vi "UHR-Fleezers Control (host) - Lorentz v3.vi"() -> ()   [LabVIEW 2014] (continued)
            n1301 = Unbundle By Name(w2020) -> ("Set 1"=w2019:dbl, "Set 2"=w2018:dbl)
            n1302 = Unbundle By Name(w2017) -> ("Set 1"=w2016:bool, "Set 2"=w2015:bool)
            n1303 = Select(t=w2013, s=w2016, f=w2019) -> (s? t:f=w2011:dbl)
            n1304 = Select(t=w2012, s=w2015, f=w2018) -> (s? t:f=w2010:dbl)
            n1305 = Bundle By Name(cluster=w2020, "Set 1"=w2011, "Set 2"=w2010) -> (w2008:cluster{"Set 1":dbl, "Set 2":dbl})
            n1306 = local write "Setpoints (V)"(w2008) -> ()
            n1307 = Multiply(x=3276.7, y=w2008) -> (x*y=w2009:cluster{"Set 1":dbl, "Set 2":dbl})
            n1308 = To Word Integer(number=w2009) -> (16bit integer=w2021:cluster{"Set 1":i16, "Set 2":i16})
          }
        }
        n1309 = Unbundle By Name(w1993) -> ("Set 1"=w1992:i16, "Set 2"=w1991:i16)
        n1310 = xnode "Read/Write Control"("FPGA VI Reference In"=w1990, "error in"=w1989, "FB Setpoint Set 1"=w1992, "FB Setpoint Set 2"=w1991) -> ("error out"=w1988:errorcluster)  [unwired: 1 out]
      }
      event "+ phase (GI)", "- phase (GI)", "+ phase (GI) 2", "- phase (GI) 2", "+ phase (RI)", "- phase (RI)", "+ phase (Green FB)", "- phase (Green FB)", "- phase (BI AO)", "+ phase (BI AO)", "- phase (BI DO)", "+ phase (BI DO)": Value Change {
        n1311 = event-data() -> ()  [unwired: 7 out]
        n1312 = Or(x="+ phase (GI)", y="- phase (GI)") -> (x .or. y?=w2057:bool)
        n1313 = Negate(x="Phase adj. (GI)") -> (-x=w2062:i16)
        n1314 = Select(t=w2062, s="+ phase (GI)", f="Phase adj. (GI)") -> (s? t:f=w2061:i16)
        n1315 = Or(x="+ phase (GI) 2", y="- phase (GI) 2") -> (x .or. y?=w2048:bool)
        n1316 = Negate(x="Phase adj. (GI) 2") -> (-x=w2053:i16)
        n1317 = Select(t=w2053, s="+ phase (GI) 2", f="Phase adj. (GI) 2") -> (s? t:f=w2049:i16)
        n1318 = Negate(x="Phase adj. (RI)") -> (-x=w2047:i16)
        n1319 = Or(x="+ phase (RI)", y="- phase (RI)") -> (x .or. y?=w2043:bool)
        n1320 = Select(t=w2047, s="+ phase (RI)", f="Phase adj. (RI)") -> (s? t:f=w2042:i16)
        n1321 = Or(x="+ phase (Green FB)", y="- phase (Green FB)") -> (x .or. y?=w2036:bool)
        n1322 = Negate(x="Phase adj. (Green FB)") -> (-x=w2041:i16)
        n1323 = Select(t=w2041, s="+ phase (Green FB)", f="Phase adj. (Green FB)") -> (s? t:f=w2037:i16)
        n1324 = Negate(x="Phase adj. (BI AO)") -> (-x=w2035:i16)
        n1325 = Or(x="+ phase (BI AO)", y="- phase (BI AO)") -> (x .or. y?=w2025:bool)
        n1326 = Select(t=w2035, s="+ phase (BI AO)", f="Phase adj. (BI AO)") -> (s? t:f=w2027:i16)
        n1327 = Negate(x="Phase adj. (BI DO)") -> (-x=w2031:i16)
        n1328 = Or(x="+ phase (BI DO)", y="- phase (BI DO)") -> (x .or. y?=w2024:bool)
        n1329 = Select(t=w2031, s="+ phase (BI DO)", f="Phase adj. (BI DO)") -> (s? t:f=w2026:i16)
        n1330 = xnode "Read/Write Control"("FPGA VI Reference In"=w2023, "Phase count adjustment (GI)"=w2061, "Phase count adjustment (GI) 2"=w2049, "Phase count adjustment (RI)"=w2042, "Phase count adjustment (Green FB)"=w2037, "Phase count adjustment (BI AO)"=w2027, "Phase count adjustment (BI D)"=w2026) -> ("FPGA VI Reference Out"=w2059:T36, "error out"=w2060:errorcluster)  [unwired: 1 in]
        n1331 = xnode "Read/Write Control"("FPGA VI Reference In"=w2059, "error in"=w2060, "+ phase (GI)"=w2057, "+ phase (GI) 2"=w2048, "+ phase (RI)"=w2043, "+ phase (Green FB)"=w2036, "+ phase (BI AO)"=w2025, "+ phase (BI D)"=w2024) -> ("error out"=w2058:errorcluster)  [unwired: 1 out]
      }
      event "Green Laser ON/OFF", "Red Laser ON/OFF", "Blue Laser ON/OFF": Value Change {
        # "This loop shouldn't be initialized.  The main 'laser ON' settings should dominate and set the others."
        n1332 = event-data() -> ()  [unwired: 7 out]
        n1333 = property on="Red Laser ON" class="Bool (strict)"("Val(Sgnl)"="Red Laser ON/OFF") -> ()  [unwired: 2 in, 2 out]
        n1334 = property on="Blue Laser ON" class="Bool (strict)"("Val(Sgnl)"="Blue Laser ON/OFF") -> ()  [unwired: 2 in, 2 out]
        n1335 = property on="Green Laser ON" class="Bool (strict)"("Val(Sgnl)"="Green Laser ON/OFF") -> ()  [unwired: 2 in, 2 out]
      }
      event "Laser interlacing mode", "Green Laser ON", "Red Laser ON", "Blue Laser ON": Value Change {
        n1336 = event-data() -> ()  [unwired: 7 out]
        n1337 = local write "Green Laser ON/OFF"("Green Laser ON") -> ()
        n1338 = local write "Blue Laser ON/OFF"("Blue Laser ON") -> ()
        n1339 = local write "Red Laser ON/OFF"("Red Laser ON") -> ()
        n1340 = case shown="False" "Green Laser ON" {
          tunnel: "Laser interlacing mode" -> [_ w2123]
          tunnel: [enum32{"Laser ON", "Laser OFF", "Interlace"}."Laser OFF" ("Green laser mode") w2123] -> w2099
          tunnel: [FALSE w2119] -> w2098
          frame False {
          }
          frame True {
            n1341 = local read "Green FB On/Off"() -> (w2120:bool)
            n1342 = Equal?(x=w2123, y=enum32{"Laser ON", "Laser OFF", "Interlace"}."Interlace") -> (x = y?=w2121:bool)
            n1343 = And(x=w2121, y=w2120) -> (x .and. y?=w2119:bool)
          }
        }
        n1344 = case shown="True" "Red Laser ON" {
          tunnel: "Laser interlacing mode" -> [_ w2116]
          tunnel: [enum32{"Laser ON", "Laser OFF", "Interlace"}."Laser OFF" ("Green laser mode") w2116] -> w2095
          tunnel: [FALSE w2112] -> w2094
          frame False {
          }
          frame True {
            n1345 = local read "Red FB On/Off"() -> (w2113:bool)
            n1346 = Equal?(x=w2116, y=enum32{"Laser ON", "Laser OFF", "Interlace"}."Interlace") -> (x = y?=w2114:bool)
            n1347 = And(x=w2114, y=w2113) -> (x .and. y?=w2112:bool)
          }
        }
        n1348 = case shown="True" "Blue Laser ON" {
          tunnel: "Laser interlacing mode" -> [_ w2107]
          tunnel: [enum32{"Laser ON", "Laser OFF", "Interlace"}."Laser OFF" ("Green laser mode") w2107] -> w2091
          tunnel: [FALSE w2105] -> w2090
          frame False {
          }
          frame True {
            n1349 = local read "Blue FB On/Off"() -> (w2106:bool)
            n1350 = Equal?(x=w2107, y=enum32{"Laser ON", "Laser OFF", "Interlace"}."Interlace") -> (x = y?=w2108:bool)
            n1351 = And(x=w2108, y=w2106) -> (x .and. y?=w2105:bool)
          }
        }
        n1352 = xnode "Read/Write Control"("FPGA VI Reference In"=w2089, "Operating Mode"=w2099, "Operating Mode 2"=w2099, "Green FB On/Off"=w2098, "Red Laser Operating Mode"=w2095, "RI Operating Mode 2"=w2095, "Red FB On/Off"=w2094, "BI Operating Mode (AO)"=w2091, "Blue Laser Operating Mode (D)"=w2091, "Blue FB On/Off"=w2090) -> ("error out"=w2100:errorcluster)  [unwired: 1 in, 1 out]
        n1353 = local read "Red FB On/Off"() -> (w2072:bool)
        n1354 = local read "Green FB On/Off"() -> (w2074:bool)
        n1355 = local read "Green Laser ON"() -> (w2073:bool)
        n1356 = local read "Red Laser ON"() -> (w2071:bool)
        n1357 = And(x=w2072, y=w2071) -> (x .and. y?=w2077:bool)
        n1358 = And(x=w2074, y=w2073) -> (x .and. y?=w2083:bool)
        n1359 = local read "Red laser intensity (V)"() -> (w2076:dbl)
        n1360 = local read "Red FB Setpoint (mV)"() -> (w2075:dbl)
        n1361 = local read "Green FB Setpoint (mV)"() -> (w2086:dbl)
        n1362 = local read "Green laser intensity (V)"() -> (w2088:dbl)
        n1363 = Multiply(x=w2076, y=1000.0) -> (x*y=w2080:dbl)
        n1364 = Subtract(x=w2075, y=5.0) -> (x-y=w2079:dbl)
        n1365 = Multiply(x=w2088, y=1000.0) -> (x*y=w2085:dbl)
        n1366 = Subtract(x=w2086, y=5.0) -> (x-y=w2084:dbl)
        n1367 = Less Or Equal?(x=w2080, y=w2079) -> (x <= y?=w2078:bool)
        n1368 = Less Or Equal?(x=w2085, y=w2084) -> (x <= y?=w2082:bool)
        n1369 = And(x=w2077, y=w2078) -> (x .and. y?=w2067:bool)
        n1370 = And(x=w2083, y=w2082) -> (x .and. y?=w2068:bool)
        n1371 = Or(x=w2068, y=w2067) -> (x .or. y?=w2066:bool)
        n1372 = case shown="True" w2066 {
          frame False {
            n1373 = local write "Laser Intensity Low (bugs to fix)"(FALSE ("Laser Intensity Low")) -> ()
          }
          frame True {
            n1374 = local write "Laser Intensity Low (bugs to fix)"(TRUE ("Laser Intensity Low")) -> ()
          }
        }
      }
      event "Invert laser interlacing": Value Change {
        n1375 = event-data() -> ()  [unwired: 7 out]
        n1376 = xnode "Read/Write Control"("FPGA VI Reference In"=w2124, "Invert GI"="Invert laser interlacing", "Invert GI 2"="Invert laser interlacing", "Invert RI"="Invert laser interlacing", "Invert RI 2"="Invert laser interlacing", "Invert BI (AO)"="Invert laser interlacing", "Invert BI (D)"="Invert laser interlacing") -> ("error out"=w2126:errorcluster)  [unwired: 1 in, 1 out]
      }
      event "Green FB Setpoint (mV)", "Green FB Gains", "Green FB On/Off", "Green Intensity % (FB OFF)", "Green int current ON count adj": Value Change {
        n1377 = event-data() -> ()  [unwired: 7 out]
        n1378 = local read "Green FB Setpoint (mV)"() -> (w2146:dbl)
        n1379 = Multiply(x=w2146, y=3.2767) -> (x*y=w2145:dbl)
        n1380 = local read "Green Intensity % (FB OFF)"() -> (w2149:dbl)
        n1381 = Multiply(x=w2149, y=655.35) -> (x*y=w2150:dbl)
        n1382 = To Unsigned Word Integer(number=w2150) -> (unsigned 16bit integer=w2148:u16)
        n1383 = local read "Green int current ON count adj"() -> (w2152:u32)
        n1384 = local read "Laser interlacing mode"() -> (w2143:enum32{"Laser ON", "Laser OFF", "Interlace"})
        n1385 = local read "Green FB Gains"() -> (w2140:T14)
        n1386 = local read "Green Laser ON"() -> (w2144:bool)
        n1387 = local read "Green FB On/Off"() -> (w2153:bool)
        n1388 = Equal?(x=w2143, y=enum32{"Laser ON", "Laser OFF", "Interlace"}."Interlace") -> (x = y?=w2141:bool)
        n1389 = Unbundle By Name(w2140) -> ("proportional gain (Kc)"=w2139:i16, "integral gain (Kc*Ts/Ti)"=w2138:i16, "derivative gain (Kc*Td/Ts)"=w2137:i16)
        n1390 = Compound Arithmetic op=AND(w2141, w2153, w2144) -> (w2127:bool)
        n1391 = local read "Green FB Setpoint (mV)"() -> (w2131:dbl)
        n1392 = local read "Green laser intensity (V)"() -> (w2134:dbl)
        n1393 = xnode "Read/Write Control"("FPGA VI Reference In"=w2136, "Green FB Setpoint"=w2145, "Green FB On/Off"=w2127, "Current Out"=w2148, "Green int current ON count adj"=w2152, "P3"=w2139, "I3"=w2138, "D3"=w2137) -> ("error out"=w2154:errorcluster)  [unwired: 1 in, 1 out]
        n1394 = Multiply(x=w2134, y=1000.0) -> (x*y=w2130:dbl)
        n1395 = Subtract(x=w2131, y=5.0) -> (x-y=w2129:dbl)
        n1396 = Less Or Equal?(x=w2130, y=w2129) -> (x <= y?=w2128:bool)
        n1397 = And(x=w2127, y=w2128) -> (x .and. y?=w2135:bool)
        n1398 = case shown="True" w2135 {
          frame False {
            n1399 = local write "Laser Intensity Low (bugs to fix)"(FALSE ("Laser Intensity Low")) -> ()
          }
          frame True {
            n1400 = local write "Laser Intensity Low (bugs to fix)"(TRUE ("Laser Intensity Low")) -> ()
          }
        }
      }
      event "Blue FB Setpoint (mV)", "Blue FB Gains", "Blue FB On/Off", "Blue Intensity % (FB OFF)", "Blue int AO ON count adjust": Value Change {
        # "Triggers blue laser serial command"
        # "16 bit analog out"
        n1401 = event-data() -> ()  [unwired: 7 out]
        n1402 = Multiply(x="Blue FB Setpoint (mV)", y=3.2767) -> (x*y=w2174:dbl)
        n1403 = Multiply(x="Blue Intensity % (FB OFF)", y=0.8) -> (x*y=w2157:dbl)
        n1404 = Number To Decimal String(number=w2157) -> (decimal integer string=w2158:string)  [unwired: 1 in]
        n1405 = Multiply(x="Blue Intensity % (FB OFF)", y=655.35) -> (x*y=w2177:dbl)
        n1406 = local write "Blue Laser Power (mW)\n(Constant Power Mode)"(w2158) -> ()
        n1407 = To Unsigned Word Integer(number=w2177) -> (unsigned 16bit integer=w2176:u16)
        n1408 = local read "Laser interlacing mode"() -> (w2172:enum32{"Laser ON", "Laser OFF", "Interlace"})
        n1409 = Unbundle By Name("Blue FB Gains") -> ("proportional gain (Kc)"=w2169:i16, "integral gain (Kc*Ts/Ti)"=w2168:i16, "derivative gain (Kc*Td/Ts)"=w2167:i16)
        n1410 = local read "Blue Laser ON"() -> (w2162:bool)
        n1411 = Equal?(x=w2172, y=enum32{"Laser ON", "Laser OFF", "Interlace"}."Interlace") -> (x = y?=w2170:bool)
        n1412 = Compound Arithmetic op=AND(w2170, "Blue FB On/Off", w2162) -> (w2173:bool)
        n1413 = xnode "Read/Write Control"("FPGA VI Reference In"=w2161, "Blue FB Setpoint"=w2174, "Blue FB On/Off"=w2173, "BI Current Out"=w2176, "Blue current ON count adj (AO)"="Blue int AO ON count adjust", "P5"=w2169, "I5"=w2168, "D5"=w2167) -> ("error out"=w2179:errorcluster)  [unwired: 1 in, 1 out]
      }
      event "Red FB Setpoint (mV)", "Red FB Gains", "Red FB On/Off", "Red Intensity % (FB OFF)": Value Change {
        n1414 = event-data() -> ()  [unwired: 7 out]
        n1415 = local read "Red FB Setpoint (mV)"() -> (w2200:dbl)
        n1416 = Multiply(x=w2200, y=3.2767) -> (x*y=w2199:dbl)
        n1417 = local read "Red Intensity % (FB OFF)"() -> (w2190:dbl)
        n1418 = Multiply(x=w2190, y=655.35) -> (x*y=w2203:dbl)
        n1419 = To Unsigned Word Integer(number=w2203) -> (unsigned 16bit integer=w2202:u16)
        n1420 = local read "Laser interlacing mode"() -> (w2197:enum32{"Laser ON", "Laser OFF", "Interlace"})
        n1421 = local read "Red FB Gains"() -> (w2194:T14)
        n1422 = local read "Red Laser ON"() -> (w2198:bool)
        n1423 = local read "Red FB On/Off"() -> (w2205:bool)
        n1424 = Equal?(x=w2197, y=enum32{"Laser ON", "Laser OFF", "Interlace"}."Interlace") -> (x = y?=w2195:bool)
        n1425 = Unbundle By Name(w2194) -> ("proportional gain (Kc)"=w2193:i16, "integral gain (Kc*Ts/Ti)"=w2192:i16, "derivative gain (Kc*Td/Ts)"=w2191:i16)
        n1426 = Compound Arithmetic op=AND(w2195, w2205, w2198) -> (w2182:bool)
        n1427 = local read "Red laser intensity (V)"() -> (w2181:dbl)
        n1428 = local read "Red FB Setpoint (mV)"() -> (w2180:dbl)
        n1429 = xnode "Read/Write Control"("FPGA VI Reference In"=w2189, "Red FB Setpoint"=w2199, "Red FB On/Off"=w2182, "RI Current Out"=w2202, "P4"=w2193, "I4"=w2192, "D4"=w2191) -> ("error out"=w2206:errorcluster)  [unwired: 1 in, 1 out]
        n1430 = Multiply(x=w2181, y=1000.0) -> (x*y=w2186:dbl)
        n1431 = Subtract(x=w2180, y=5.0) -> (x-y=w2185:dbl)
        n1432 = Less Or Equal?(x=w2186, y=w2185) -> (x <= y?=w2184:bool)
        n1433 = And(x=w2182, y=w2184) -> (x .and. y?=w2183:bool)
        n1434 = case shown="False" w2183 {
          frame False {
            n1435 = local write "Laser Intensity Low (bugs to fix)"(FALSE ("Laser Intensity Low")) -> ()
          }
          frame True {
            n1436 = local write "Laser Intensity Low (bugs to fix)"(TRUE ("Laser Intensity Low")) -> ()
          }
        }
      }
      event "+ phase (APD 1 Gate)", "- phase (APD 1 Gate)", "+ phase (APD 2 Gate)", "- phase (APD 2 Gate)", "+ phase (APD 3 Gate)", "- phase (APD 3 Gate)", "+ phase (APD Acq)", "- phase (APD Acq)": Value Change {
        n1437 = event-data() -> ()  [unwired: 7 out]
        n1438 = local read "Phase Adj. (APD 1 Gate)"() -> (w2229:i16)
        n1439 = Or(x="- phase (APD 1 Gate)", y="+ phase (APD 1 Gate)") -> (x .or. y?=w2231:bool)
        n1440 = Negate(x=w2229) -> (-x=w2236:i16)
        n1441 = Select(t=w2236, s="+ phase (APD 1 Gate)", f=w2229) -> (s? t:f=w2235:i16)
        n1442 = local read "Phase Adj. (APD 2 Gate)"() -> (w2226:i16)
        n1443 = Or(x="- phase (APD 2 Gate)", y="+ phase (APD 2 Gate)") -> (x .or. y?=w2224:bool)
        n1444 = Negate(x=w2226) -> (-x=w2228:i16)
        n1445 = Select(t=w2228, s="+ phase (APD 2 Gate)", f=w2226) -> (s? t:f=w2225:i16)
        n1446 = Negate(x="Phase Adj. (APD 3 Gate)") -> (-x=w2223:i16)
        n1447 = Or(x="- phase (APD 3 Gate)", y="+ phase (APD 3 Gate)") -> (x .or. y?=w2219:bool)
        n1448 = Select(t=w2223, s="+ phase (APD 3 Gate)", f="Phase Adj. (APD 3 Gate)") -> (s? t:f=w2220:i16)
        n1449 = local read "Phase Adj. (APD Acq)"() -> (w2217:i16)
        n1450 = Or(x="- phase (APD Acq)", y="+ phase (APD Acq)") -> (x .or. y?=w2215:bool)
        n1451 = Negate(x=w2217) -> (-x=w2218:i16)
        n1452 = Select(t=w2218, s="+ phase (APD Acq)", f=w2217) -> (s? t:f=w2216:i16)
        n1453 = xnode "Read/Write Control"("FPGA VI Reference In"=w2209, "Phase count adjustment (APD 1 Gate)"=w2235, "Phase count adjustment (APD 2 Gate)"=w2225, "Phase count adjustment (APD 3 Gate)"=w2220, "Phase Count Adjustment (APD Acq)"=w2216) -> ("FPGA VI Reference Out"=w2233:T36, "error out"=w2234:errorcluster)  [unwired: 1 in]
        n1454 = xnode "Read/Write Control"("FPGA VI Reference In"=w2233, "error in"=w2234, "+ phase (APD 1 Gate)"=w2231, "+ phase (APD 2 Gate)"=w2224, "+ phase (APD 3 Gate)"=w2219, "+ phase (APD Acq)"=w2215) -> ("error out"=w2232:errorcluster)  [unwired: 1 out]
      }
      event "Invert APD Gate", "APD Gate ON Count", "APD Gate OFF Count", "APD Gate", "APD Integration Time (s)", "APD AO Scale Factor", "Duty Frequency (ON 1/N cycles)", "Interlace ON count", "Interlace OFF count": Value Change {
        n1455 = event-data() -> ()  [unwired: 7 out]
        n1456 = Add(x="Interlace ON count", y="Interlace OFF count") -> (x+y=w2243:u16)
        n1457 = Add(x="APD Gate ON Count", y="APD Gate OFF Count") -> (x+y=w2254:u16)
        n1458 = Multiply(x="Duty Frequency (ON 1/N cycles)", y=w2243) -> (x*y=w2239:u16)
        "Green AI Count" <- w2239
        "Red AI Count" <- w2239
        "Blue AI Count" <- w2239
        n1459 = Subtract(x=w2239, y="Interlace ON count") -> (x-y=w2242:u16)
        n1460 = Multiply(x=w2254, y="Duty Frequency (ON 1/N cycles)") -> (x*y=w2253:u16)
        n1461 = Subtract(x=w2253, y="APD Gate ON Count") -> (x-y=w2252:u16)
        n1462 = local read "DMA Update Period (s)"() -> (w2255:dbl)
        n1463 = Multiply(x="APD Integration Time (s)", y=40000000.0) -> (x*y=w2259:dbl)
        n1464 = Reciprocal(x="APD Integration Time (s)") -> (1/x=→"APD Acq Rate (Hz)":dbl)
        n1465 = To Unsigned Long Integer(number=w2259) -> (unsigned 32bit integer=w2245:u32)
        "APD Int. Count" <- w2245
        n1466 = local read "Number of APDs"() -> (w2238:u8)
        n1467 = Divide(x=w2255, y="APD Integration Time (s)") -> (x/y=w2257:dbl)
        n1468 = Multiply(x=w2238, y=w2257) -> (x*y=w2256:dbl)
        n1469 = local write "APD Samples/FIFO Acq."(w2257) -> ()
        n1470 = local write "APD Elements/DMA read"(w2256) -> ()
        n1471 = xnode "Read/Write Control"("FPGA VI Reference In"=w2237, "Invert APD Gate"="Invert APD Gate", "APD Gate ON Count"="APD Gate ON Count", "APD Gate OFF Count"=w2252, "APD Acq Rate Count"=w2245, "APD Gate Operating Mode"="APD Gate", "APD AO scale factor"="APD AO Scale Factor", "Green interlace ON count"="Interlace ON count", "Green interlace OFF count"=w2242, "Green interlace ON count 2"="Interlace ON count", "Green interlace OFF count 2"=w2242, "Green FB Count"=w2239, "Red interlace ON count"="Interlace ON count", "Red interlace OFF count"="Interlace OFF count", "Blue ON count (AO)"="Interlace ON count", "Blue OFF count (AO)"="Interlace OFF count", "Blue interlace OFF count (D)"="Interlace OFF count", "Blue interlace ON count (D)"="Interlace ON count") -> ("error out"=w2261:errorcluster)  [unwired: 1 in, 1 out]
      }
      event "Neg. TTrig FPGA": Value Change {
        n1472 = event-data() -> ()  [unwired: 7 out]
        n1473 = xnode "Read/Write Control"("FPGA VI Reference In"=w2262, "TTrig Negate Pos"="Neg. TTrig FPGA") -> ()  [unwired: 1 in, 2 out]
      }
      event "Test ttrig": Value Change {
        n1474 = event-data() -> ()  [unwired: 7 out]
        n1475 = xnode "Read/Write Control"("FPGA VI Reference In"=w2264, "TTrig?"=TRUE) -> ("error out"=w2266:errorcluster)  [unwired: 1 in, 1 out]
      }
      event "Number of F/B Scans (AOD)", "Scan Speed (nm/s)", "Scan BD", "Initial delta (MHz)", "Step Size (nm)", "Scan Range (nm)": Value Change {
        w2330 = 123.0  # AOM cal (nm/MHz)
        n1476 = event-data() -> ()  [unwired: 7 out]
        n1477 = local read "BD 1 Frequency 1 (MHz)"() -> (w2313:dbl)
        n1478 = local read "AOM X Cal (nm/MHz)"() -> (w2305:dbl)
        n1479 = local read "X RF Frequency Limits (MHz)"() -> (w2317:T24)
        n1480 = local read "Y RF Frequency Limits (MHz)"() -> (w2314:T24)
        n1481 = local read "BD 2 Frequency 1 (MHz)"() -> (w2319:dbl)
        n1482 = Negate(x="Scan Range (nm)") -> (-x=w2283:dbl)
        n1483 = Divide(x=w2283, y=w2305) -> (x/y=w2287:dbl)
        n1484 = Select(t=w2317, s="Scan BD", f=w2314) -> (s? t:f=w2316:T24)
        n1485 = Select(t=w2313, s="Scan BD", f=w2319) -> (s? t:f=w2318:dbl)
        n1486 = Unbundle By Name(w2316) -> ("Maximum"=w2325:dbl, "Minimum"=w2324:dbl)
        n1487 = Add(x=w2287, y=w2318) -> (x+y=w2322:dbl)
        n1488 = Divide(x=w2283, y="Step Size (nm)") -> (x/y=w2302:dbl)
        n1489 = Divide(x="Step Size (nm)", y=w2305) -> (x/y=w2311:dbl)
        n1490 = Absolute Value(x=w2302) -> (abs(x)=w2286:dbl)
        n1491 = Sign(1:w2283) -> (0:w2284:dbl)
        n1492 = In Range and Coerce(upper limit=w2325, x=w2322, lower limit=w2324) -> (coerced(x)=w2321:dbl, In Range?=w2323:bool)
        n1493 = To Unsigned Quad Integer(1:w2286) -> (0:w2301:u64)
        "Scan steps (AOD)" <- w2301
        n1494 = call "IR AOM freq to word.vi"("Frequency In (MHz)"=w2311) -> ("Frequency Word Out (double)"=w2308:dbl)
        n1495 = Multiply(x=w2284, y=w2308) -> (x*y=w2285:dbl)
        n1496 = Subtract(x=w2322, y=w2321) -> (x-y=w2320:dbl)
        n1497 = To Quad Integer(1:w2285) -> (0:w2307:i64)
        "Incr. int (AOD)" <- w2307
        n1498 = Subtract(x=w2287, y=w2320) -> (x-y=w2306:dbl)
        "Scan Range (MHz)" <- w2306
        n1499 = Select(t=w2287, s=w2323, f=w2306) -> (s? t:f=w2326:dbl)
        n1500 = Multiply(x=w2306, y=w2305) -> (x*y=w2304:dbl)
        n1501 = Decrement(x=w2301) -> (x-1=w2354:u64)
        n1502 = Negate(x=w2304) -> (-x=w2300:dbl)
        n1503 = local write "Scan Range (nm)"(w2300) -> ()
        n1504 = Divide(x=w2326, y=w2354) -> (x/y=w2310:dbl)
        "Scan Increment (MHz)" <- w2310
        n1505 = call "IR AOM freq to word.vi"("Frequency In (MHz)"=w2310) -> ("Frequency Word Out (double)"=w2309:dbl)
        n1506 = Divide(x="Step Size (nm)", y="Scan Speed (nm/s)") -> (x/y=w2297:dbl)
        n1507 = To Quad Integer(1:w2309) -> ()  [unwired: 1 out]
        n1508 = local read "Number Interlace Sets"() -> (w2281:u8)
        n1509 = local read "AI Count (ticks)"() -> (w2282:u16)
        n1510 = local read "Total Counts (ticks)"() -> (w2280:u16)
        n1511 = local read "# Samples/trap"() -> (w2312:u32)
        n1512 = Multiply(x=w2282, y=w2281) -> (x*y=w2279:u16)
        n1513 = Divide(x=w2280, y=w2279) -> (x/y=w2278:dbl)
        n1514 = Select(t=w2313, s="Scan BD", f=w2319) -> (s? t:f=w2351:dbl)
        "Initial freq. (MHz)" <- w2351
        n1515 = Add(x=w2326, y=w2351) -> (x+y=→"Final freq. (MHz)":dbl)
        n1516 = Divide(x=w2280, y=40000000.0) -> (x/y=w2296:dbl)
        n1517 = Divide(x=w2297, y=w2296) -> (x/y=w2295:dbl)
        n1518 = To Unsigned Quad Integer(1:w2295) -> (0:w2270:u64)
        n1519 = Quotient & Remainder(x=w2270, y=u64 2) -> (x-y*floor(x/y)=w2274:u64)  [unwired: 1 out]
        n1520 = Equal?(x=w2274, y=u64 0) -> (x = y?=w2272:bool)
        n1521 = Decrement(x=w2270) -> (x-1=w2271:u64)
        n1522 = Select(t=w2270, s=w2272, f=w2271) -> (s? t:f=w2269:u64)
        "Cycles/step (AOD)" <- w2269
        n1523 = xnode "Read/Write Control"("FPGA VI Reference In"=w2268, "Scan steps"=w2301, "Number of scans"="Number of F/B Scans (AOD)", "Cycles per step"=w2269, "Scan freq.  increment"=w2307, "Scan BD"="Scan BD") -> ("error out"=w2360:errorcluster)  [unwired: 1 in, 1 out]
        n1524 = Multiply(x=w2301, y=w2269) -> (x*y=w2355:u64)
        n1525 = Multiply(x=w2355, y=u64 2) -> (x*y=w2277:u64)
        n1526 = Multiply(x=w2278, y=w2277) -> (x*y=w2276:dbl)
        "Data points/scan (f/b)" <- w2276
        n1527 = Multiply(x=w2276, y="Number of F/B Scans (AOD)") -> (x*y=w2358:dbl)
        "Data points/scans" <- w2358
        n1528 = Divide(x=w2358, y=w2312) -> (x/y=→"N sets should be saved":dbl)
        n1529 = Multiply(x=w2355, y=w2296) -> (x*y=w2294:dbl)
        "Time/Scan (s) (AOD)" <- w2294
        n1530 = Select(t=w2326, s="Scan BD", f=0.0) -> (s? t:f=w2352:dbl)
        n1531 = Select(t=0.0, s="Scan BD", f=w2326) -> (s? t:f=w2348:dbl)
        n1532 = local read "BD 2 Frequency 2 (MHz)"() -> (w2344:dbl)
        n1533 = local read "BD 1 Frequency 2 (MHz)"() -> (w2347:dbl)
        n1534 = Add(x=w2348, y=w2319) -> (x+y=w2345:dbl)
        n1535 = Add(x=w2313, y=w2352) -> (x+y=w2346:dbl)
        n1536 = Multiply(x=w2294, y=2.0) -> (x*y=w2293:dbl)
        n1537 = Multiply(x=w2293, y="Number of F/B Scans (AOD)") -> (x*y=w2290:dbl)
        n1538 = Divide(x=w2290, y=60.0) -> (x/y=→"Time to Finish All (min)":dbl)
        n1539 = Add(x="Trap 2 Bead Size (nm)", y="Trap 1 Bead Size (nm)") -> (x+y=w2334:dbl)
        n1540 = Divide(x=w2334, y=2.0) -> (x/y=w2328:dbl)
        n1541 = local read "Initial delta (MHz)"() -> (w2331:dbl)
        n1542 = Subtract(x=w2345, y=w2344) -> (x-y=w2342:dbl)
        n1543 = Subtract(x=w2346, y=w2347) -> (x-y=w2343:dbl)
        n1544 = Square(x=w2342) -> (x^2=w2341:dbl)
        n1545 = Square(x=w2343) -> (x^2=w2340:dbl)
        n1546 = Add(x=w2340, y=w2341) -> (x+y=w2339:dbl)
        n1547 = Square Root(x=w2339) -> (sqrt(x)=w2338:dbl)
        "Final delta (MHz)" <- w2338
        n1548 = Multiply(x=w2330, y=w2338) -> (x*y=w2337:dbl)
        n1549 = Multiply(x=w2331, y=w2330) -> (x*y=w2329:dbl)
        n1550 = Subtract(x=w2329, y=w2328) -> (x-y=→"Initial sep (nm)":dbl)
        n1551 = Subtract(x=w2337, y=w2328) -> (x-y=→"Final sep (nm)":dbl)
      }
      event "Freq or Amp switch first", "Swap F1 and F2", "Freq switch delay", "Amp switch delay": Value Change {
        n1552 = event-data() -> ()  [unwired: 7 out]
        n1553 = local read "Amp switch delay"() -> (w2362:u16)
        n1554 = local read "Swap F1 and F2"() -> (w2363:bool)
        n1555 = xnode "Read/Write Control"("FPGA VI Reference In"=w2361, "Swap F1 and F2"=w2363, "Amp switch delay"=w2362) -> ("error out"=w2364:errorcluster)  [unwired: 1 in, 1 out]
      }
      event "Scan steps (MCL)", "Number of scans (MCL)", "Scan Range (V)\n(of steps)", "2D or 1D Scan", "N APD Samp/step", "Fast Scan Dir", "Continuous MCL Scanning", "Scan lines (y)": Value Change {
        w2367 = 32767.0 ("y")
        n1556 = event-data() -> ()  [unwired: 7 out]
        n1557 = Select(t="Scan lines (y)", s="2D or 1D Scan", f="Number of scans (MCL)") -> (s? t:f=w2372:u64)
        n1558 = Decrement(x="Scan steps (MCL)") -> (x-1=w2388:u64)
        n1559 = Divide(x="Scan Range (V)\n(of steps)", y=w2388) -> (x/y=w2387:dbl)
        "Desired Scan Incr (V)" <- w2387
        n1560 = local read "APD Integration Time (s)"() -> (w2380:dbl)
        n1561 = Multiply(x=w2387, y=w2367) -> (x*y=w2396:dbl)
        n1562 = Divide(x=w2396, y=10.0) -> (x/y=w2386:dbl)
        "Desired incr (int)" <- w2386
        n1563 = local read "Update Count (MCL)"() -> (w2392:u32)
        n1564 = Round Toward -Infinity(1:w2386) -> (0:w2395:dbl)
        n1565 = To Word Integer(number=w2395) -> (16bit integer=w2370:i16)
        "Actual Incr. int (MCL)" <- w2370
        n1566 = Multiply(x=w2380, y=40000000.0) -> (x*y=w2393:dbl)
        n1567 = Divide(x=w2393, y=w2392) -> (x/y=w2391:dbl)
        n1568 = Multiply(x=i16 10, y=w2370) -> (x*y=w2368:i16)
        n1569 = Multiply(x="N APD Samp/step", y=w2391) -> (x*y=w2390:dbl)
        "Cycles/step (MCL)" <- w2390
        n1570 = Divide(x=w2368, y=w2367) -> (x/y=→"Actual MCL Inc (V)":dbl)
        n1571 = Multiply(x="N APD Samp/step", y="Scan steps (MCL)") -> (x*y=w2382:dbl)
        n1572 = local read "APD Samples/FIFO Acq."() -> (w2379:dbl)
        n1573 = Multiply(x=w2382, y=u64 2) -> (x*y=w2381:dbl)
        "Data points/scan (f+b)" <- w2381
        n1574 = Multiply(x=w2381, y=w2372) -> (x*y=w2399:dbl)
        "Data points/scans (MCL)" <- w2399
        n1575 = Multiply(x=w2380, y=w2381) -> (x*y=w2373:dbl)
        "Time/f+b scan (s) (MCL)" <- w2373
        n1576 = Divide(x=w2399, y=w2379) -> (x/y=→"N sets should be saved (MCL)":dbl)
        n1577 = Multiply(x=w2373, y=w2372) -> (x*y=→"Total Time (s)":dbl)
        n1578 = Not(x="Fast Scan Dir") -> (.not. x?=w2377:bool)
        n1579 = xnode "Read/Write Control"("FPGA VI Reference In"=w2365, "Scan steps (MCL)"="Scan steps (MCL)", "Number of scans (MCL)"=w2372, "Cycles per step (MCL)"=w2390, "Scan freq.  increment (MCL)"=w2370, "1D or 2D Scan?"="2D or 1D Scan", "MCL Scan Axis"=w2377, "Cont. Scan (MCL)"="Continuous MCL Scanning") -> ("error out"=w2401:errorcluster)  [unwired: 1 in, 1 out]
      }
      event "Read Cal": Value Change {
        w2440 = 1000.0 ("y")
        w2423 = T45."big-endian, network order" ("byte order (0:big-endian, network order)")
        w2424 = -1 ("count (1)")
        n1580 = event-data() -> ()  [unwired: 7 out]
        n1581 = local read "Save file name"() -> (w2456:path)
        n1582 = local write "Read Cal"(FALSE ("Read Cal")) -> ()
        n1583 = Strip Path(path=w2456) -> (stripped path=w2455:path)  [unwired: 1 out]
        n1584 = Path To String(path=w2455) -> (string=w2432:string)
        n1585 = Concatenate Strings(w2432, "\\current.cal" ("string")) -> (w2453:string)
        n1586 = Concatenate Strings(w2432, "\\current.off" ("string")) -> (w2430:string)
        n1587 = String To Path(string=w2453) -> (path=w2452:path)
        n1588 = String To Path(string=w2430) -> (path=w2427:path)
        n1589 = Open/Create/Replace File(file path (use dialog)=w2452, operation (0:open)=T44."open", access (0:read/write)=enum16{"read/write", "read-only", "write-only"}."read-only") -> (refnum out=w2459:refnum<file>, error out=w2448:errorcluster)  [unwired: 1 in, 3 out]
        n1590 = Open/Create/Replace File(file path (use dialog)=w2427, operation (0:open)=T44."open", access (0:read/write)=enum16{"read/write", "read-only", "write-only"}."read-only") -> (refnum out=w2426:refnum<file>)  [unwired: 1 in, 4 out]
        n1591 = Deny Access(4:w2448, 7:w2459) -> (0:w2447:errorcluster, 3:w2451:refnum<file>)  [unwired: 1 out]
        n1592 = Deny Access(7:w2426) -> (3:w2425:refnum<file>)  [unwired: 1 in, 2 out]
        n1593 = Read from Binary File(5:0.0, 8:w2447, 9:w2423, 10:w2424, 11:w2451) -> (0:w2446:errorcluster, 2:w2444:dbl[], 3:w2449:refnum<file>)  [unwired: 2 out]
        n1594 = Array To Cluster(array=w2444) -> (cluster=w2443:T47)
        n1595 = Unbundle(w2443) -> ("[0]"=w2411:dbl, "[1]"=w2409:dbl, "[2]"=w2410:dbl, "[3]"=w2408:dbl, "[4]"=w2442:dbl, "[5]"=w2441:dbl)
        n1596 = Close File(refnum=w2449, error in=w2446) -> (error out=→"Read cal error":errorcluster)  [unwired: 1 out]
        n1597 = Multiply(x=w2442, y=w2440) -> (x*y=w2437:dbl)
        n1598 = Multiply(x=w2441, y=w2440) -> (x*y=w2433:dbl)
        n1599 = Read from Binary File(5:0.0, 9:w2423, 10:w2424, 11:w2425) -> (2:w2419:dbl[], 3:w2417:refnum<file>)  [unwired: 1 in, 3 out]
        n1600 = Close File(refnum=w2417) -> ()  [unwired: 1 in, 2 out]
        n1601 = Bundle By Name(cluster="T1 calibration", "T1 alpha_x (nm/V)"=w2411, "T1 offset_x (mV)"=w2437, "T1 kappa_x (pN/nm)"=w2410) -> (w2436:T9)
        n1602 = Array Subset(array=w2419, index=1) -> (w2416:dbl[])  [unwired: 1 in]
        n1603 = Bundle By Name(cluster="T2 calibration", "T2 alpha_x (nm/V)"=w2409, "T2 offset_x (mV)"=w2433, "T2 kappa_x (pN/nm)"=w2408) -> (w2434:T8)
        n1604 = Index Array(array=w2419, index=0) -> (element=→"Offset file step size":dbl)
        n1605 = local write "T1 calibration"(w2436) -> ()
        n1606 = local write "T2 calibration"(w2434) -> ()
        n1607 = Decimate 1D Array(w2416) -> (w2406:dbl[], w2405:dbl[])  [unwired: 1 out]
        n1608 = Multiply(x=w2411, y=w2410) -> (x*y=w2412:dbl)
        n1609 = Multiply(x=w2409, y=w2408) -> (x*y=w2413:dbl)
        n1610 = Divide(x=w2413, y=w2412) -> (x/y=w2404:dbl)
        n1611 = property on="B factor" class="DigNum (strict)"("Val(Sgnl)"=w2404) -> ()  [unwired: 2 in, 2 out]
        n1612 = Bundle By Name(cluster="Offset Values", "Trap 1X offset"=w2406, "Trap 2X offset"=w2405) -> (w2414:T20)
        n1613 = Multiply(x=w2405, y=w2404) -> (x*y=w2407:dbl[])
        n1614 = local write "Offset Values"(w2414) -> ()
        n1615 = Subtract(x=w2406, y=w2407) -> (x-y=w2402:dbl[])
        n1616 = case shown="True" "Auto read offset correction" {
          tunnel: w2402 -> [_ w2460]
          frame False {
          }
          frame True {
            n1617 = property on="Setpoint offset\ncorrection values" class="Arr (strict)"("Val(Sgnl)"=w2460) -> ()  [unwired: 2 in, 2 out]
          }
        }
      }
      event "Abort MCL Scan": Value Change {
        n1618 = event-data() -> ()  [unwired: 7 out]
        n1619 = local write "MCL Scanning"(FALSE ("MCL Scanning")) -> ()
        n1620 = xnode "Read/Write Control"("FPGA VI Reference In"=w2461, "Abort scan (MCL)"="Abort MCL Scan") -> ("error out"=w2464:errorcluster)  [unwired: 1 in, 1 out]
      }
      event "Update Count (MCL)": Value Change {
        n1621 = event-data() -> ()  [unwired: 7 out]
        n1622 = xnode "Read/Write Control"("FPGA VI Reference In"=w2465, "MCL count"="Update Count (MCL)") -> ("error out"=w2467:errorcluster)  [unwired: 1 in, 1 out]
      }
      event "+ phase (MCL)", "- phase (MCL)": Value Change {
        n1623 = event-data() -> ()  [unwired: 7 out]
        n1624 = Or(x="- phase (MCL)", y="+ phase (MCL)") -> (x .or. y?=w2471:bool)
        n1625 = Negate(x="Phase adjust (MCL)") -> (-x=w2477:i16)
        n1626 = Select(t=w2477, s="+ phase (MCL)", f="Phase adjust (MCL)") -> (s? t:f=w2475:i16)
        n1627 = xnode "Read/Write Control"("FPGA VI Reference In"=w2468, "Phase count adjustment (MCL)"=w2475) -> ("FPGA VI Reference Out"=w2472:T36, "error out"=w2473:errorcluster)  [unwired: 1 in]
        n1628 = xnode "Read/Write Control"("FPGA VI Reference In"=w2472, "error in"=w2473, "+ phase (MCL)"=w2471) -> ("error out"=w2470:errorcluster)  [unwired: 1 out]
      }
      event "Abort AOD Scan": Value Change {
        n1629 = event-data() -> ()  [unwired: 7 out]
        n1630 = xnode "Read/Write Control"("FPGA VI Reference In"=w2478, "Abort scan"="Abort AOD Scan") -> ("error out"=w2480:errorcluster)  [unwired: 1 in, 1 out]
      }
      event "Continuous AOD Scanning": Value Change {
        n1631 = event-data() -> ()  [unwired: 7 out]
        n1632 = xnode "Read/Write Control"("FPGA VI Reference In"=w2481, "Cont. Scan"="Continuous AOD Scanning") -> ("error out"=w2483:errorcluster)  [unwired: 1 in, 1 out]
      }
      event "Index": Value Change {
        n1633 = event-data() -> ()  [unwired: 7 out]
        n1634 = call "Create new save file.vi"("Insert"="", "Ext"=".dat" ("string"), "Index In"="Index") -> ("Path Out"=→"Save file name":path, "Index Out"=w2484:dbl)
        "Save index" <- w2484
        n1635 = local write "Index"(w2484) -> ()
      }
      event "AO1", "AO2": Value Change {
        w2498 = 10.0 ("y")
        w2497 = 32767.0 ("y")
        n1636 = event-data() -> ()  [unwired: 7 out]
        n1637 = local read "AO2"() -> (w2496:dbl)
        n1638 = local read "AO1"() -> (w2493:dbl)
        n1639 = Multiply(x=w2493, y=w2497) -> (x*y=w2492:dbl)
        n1640 = Multiply(x=w2496, y=w2497) -> (x*y=w2495:dbl)
        n1641 = Divide(x=w2492, y=w2498) -> (x/y=w2491:dbl)
        n1642 = Divide(x=w2495, y=w2498) -> (x/y=w2494:dbl)
        n1643 = To Word Integer(number=w2491) -> (16bit integer=w2499:i16)
        n1644 = To Word Integer(number=w2494) -> (16bit integer=w2500:i16)
        n1645 = xnode "Read/Write Control"("FPGA VI Reference In"=w2489, "AO1"=w2499, "AO2"=w2500) -> ("error out"=w2490:errorcluster)  [unwired: 1 in, 1 out]
      }
      event "Inject Pump 1": Value Change {
        n1646 = event-data() -> ()  [unwired: 7 out]
        n1647 = disable-structure shown="Disabled" {
          disable-tunnel: w2501 -> [w2502 _]
          frame Disabled {
            n1648 = local read "Use Harvard pumps\nfor beads (else Chemyx)"() -> (w2503:bool)
            n1649 = case shown="True" w2503 {
              tunnel: "Inject Pump 1" -> [w2507 w2548]
              tunnel: w2502 -> [_ w2549]
              frame False {
                n1650 = local read "Pump write delay (ms)"() -> (w2506:dbl)
                n1651 = local read "Chemyx Syringe Pump Serial Port"() -> (w2505:refnum<visa-resource-name>)
                n1652 = case shown="True" w2507 {
                  tunnel: w2506 -> [w2513 w2527]
                  tunnel: w2505 -> [w2510 w2526]
                  frame False {
                    n1653 = flat-sequence {
                      tunnel: w2510 -> [w2514]
                      tunnel: [w2514] -> w2511
                      tunnel: w2513 -> [_]
                      tunnel: [w2517] -> w2512
                      tunnel: w2511 -> [w2517]
                      tunnel: w2512 -> [w2518]
                      tunnel: [w2518] -> w2508
                      tunnel: [w2520] -> w2509
                      tunnel: w2508 -> [w2520]
                      tunnel: w2509 -> [w2522]
                      frame #0 {
                        n1654 = call "Write to pump.vi"("string"="enter pump1", "VISA resource name"=w2514) -> ()  [unwired: 1 out]
                      }
                      frame #1 {
                        n1655 = Wait (ms)(milliseconds to wait="Pump pause delay (ms)") -> ()  [unwired: 1 out]
                      }
                      frame #2 {
                        n1656 = call "Write to pump.vi"("string"="stop", "VISA resource name"=w2518) -> ()  [unwired: 1 out]
                      }
                      frame #3 {
                        n1657 = Wait (ms)(milliseconds to wait=u32 500) -> ()  [unwired: 1 out]
                      }
                      frame #4 {
                        n1658 = call "Write to pump.vi"("string"="stop", "VISA resource name"=w2522) -> ()  [unwired: 1 out]
                      }
                    }
                  }
                  frame True {
                    n1659 = flat-sequence {
                      tunnel: w2526 -> [w2536]
                      tunnel: w2527 -> [w2531]
                      tunnel: w2527 -> [w2538]
                      tunnel: w2526 -> [w2539]
                      tunnel: [w2539] -> w2524
                      tunnel: [w2541] -> w2525
                      tunnel: w2524 -> [w2541]
                      tunnel: w2525 -> [w2543]
                      frame #0 {
                        n1660 = local read "All Pump Parameters"() -> (w2530:T10)
                        n1661 = Unbundle By Name(w2530) -> ("Pump 1"=w2537:T48)
                        n1662 = call "Set pump parameters.vi"("Pump write delay (ms)"=w2531, "Volume (uL)"="Ch 1 Inject Volume (uL)", "Rate (uL/h)"="Ch 1 Inject Rate (ul/h)", "Units"=4.0, "Pump #"=1.0, "Pump Parameters In"=w2537, "VISA resource name"=w2536) -> ("Pump Parameters Out"=w2529:T48)  [unwired: 3 in]
                        n1663 = Bundle By Name(cluster=w2530, "Pump 1"=w2529) -> (w2528:T10)
                        n1664 = local write "All Pump Parameters"(w2528) -> ()
                      }
                      frame #1 {
                        n1665 = Wait (ms)(milliseconds to wait=w2538) -> ()  [unwired: 1 out]
                      }
                      frame #2 {
                        n1666 = call "Write to pump.vi"("string"="start", "VISA resource name"=w2539) -> ()  [unwired: 1 out]
                      }
                      frame #3 {
                        n1667 = Wait (ms)(milliseconds to wait=u32 500) -> ()  [unwired: 1 out]
                      }
                      frame #4 {
                        n1668 = call "Write to pump.vi"("string"="start", "VISA resource name"=w2543) -> ()  [unwired: 1 out]
                      }
                    }
                  }
                }
              }
              frame True {
                n1669 = case shown="False" w2548 {
                  tunnel: w2549 -> [w2561 w2571]
                  frame False {
                    n1670 = flat-sequence {
                      tunnel: w2561 -> [w2563]
                      frame #0 {
                        n1671 = local write "Flushing P1"(FALSE ("Flushing P1")) -> ()
                        n1672 = Concatenate Strings("stop" ("string"), "\r") -> (w2565:string)
                        n1673 = VISA Write(VISA resource name=w2563, write buffer=w2565) -> ()  [unwired: 1 in, 3 out]
                      }
                      frame #1 {
                        n1674 = property on="Clear Volume P1" class="Bool (strict)"("Val(Sgnl)"=TRUE ("Value (Signaling)")) -> ()  [unwired: 2 in, 2 out]
                      }
                    }
                  }
                  frame True {
                    n1675 = local read "Normal Flow Rate (ul/h) P1"() -> (w2569:dbl)
                    n1676 = Number To Decimal String(number=w2569) -> (decimal integer string=w2575:string)  [unwired: 1 in]
                    n1677 = Concatenate Strings("irate  " ("string"), w2575, " u/h" ("string"), "\r") -> (w2573:string)
                    n1678 = VISA Write(VISA resource name=w2571, write buffer=w2573) -> (VISA resource name out=w2570:refnum<visa-resource-name>)  [unwired: 1 in, 2 out]
                    n1679 = Concatenate Strings("irun" ("string"), "\r") -> (w2577:string)
                    n1680 = VISA Write(VISA resource name=w2570, write buffer=w2577) -> ()  [unwired: 1 in, 3 out]
                  }
                }
                n1681 = local read "Saving..."() -> (w2546:bool)
                n1682 = local read "Save Event Log?"() -> (w2545:bool)
                n1683 = And(x=w2546, y=w2545) -> (x .and. y?=w2547:bool)
                n1684 = case shown="True" w2547 {
                  tunnel: w2548 -> [_ w2559]
                  frame False {
                  }
                  frame True {
                    n1685 = local read "Normal Flow Rate (ul/h) P1"() -> (w2550:dbl)
                    n1686 = Number To Decimal String(number=w2550) -> (decimal integer string=w2551:string)  [unwired: 1 in]
                    n1687 = Concatenate Strings("on, flow rate", w2551) -> (w2553:string)
                    n1688 = Select(t=w2553, s=w2559, f="off") -> (s? t:f=w2555:string)
                    n1689 = local read "log file ref"() -> (w2560:refnum<file>)
                    n1690 = local read "Time (s)"() -> (w2554:dbl)
                    n1691 = Concatenate Strings("pump 1 ", w2555) -> (w2557:string)
                    n1692 = call "write to event log.vi"("log file ref"=w2560, "time"=w2554, "input string"=w2557) -> ()  [unwired: 8 in]
                  }
                }
              }
            }
          }
          frame Enabled {
          }
        }
      }
      event "Inject Top:": Value Change {
        n1693 = event-data() -> ()  [unwired: 7 out]
        n1694 = call "hamilton_controller.vi"("Open?"="Inject Top:", "valve"=enum16{"A", "B", "C", "D", "ALL"}."A", "action"=T42."MOVE VALVE") -> ("error out"=w2579:errorcluster)  [unwired: 7 in, 1 out]
      }
      event "Inject Bottom:": Value Change {
        n1695 = event-data() -> ()  [unwired: 7 out]
        n1696 = call "hamilton_controller.vi"("Open?"="Inject Bottom:", "valve"=enum16{"A", "B", "C", "D", "ALL"}."B", "action"=T42."MOVE VALVE") -> ("error out"=w2583:errorcluster)  [unwired: 7 in, 1 out]
      }
      event "Inject Main:": Value Change {
        n1697 = event-data() -> ()  [unwired: 7 out]
        n1698 = call "hamilton_controller.vi"("Open?"="Inject Main:", "valve"=enum16{"A", "B", "C", "D", "ALL"}."C", "action"=T42."MOVE VALVE") -> ("error out"=w2587:errorcluster)  [unwired: 7 in, 1 out]
      }
      event "Inject Pump 3": Value Change {
        n1699 = event-data() -> ()  [unwired: 7 out]
        n1700 = local read "Use Harvard pumps\nfor beads (else Chemyx)"() -> (w2592:bool)
        n1701 = disable-structure shown="Disabled" {
          disable-tunnel: w2592 -> [w2594 _]
          disable-tunnel: w2591 -> [w2593 _]
          frame Disabled {
            n1702 = case shown="True" w2594 {
              tunnel: "Inject Pump 3" -> [w2598 w2639]
              tunnel: w2593 -> [_ w2640]
              frame False {
                n1703 = local read "Pump write delay (ms)"() -> (w2597:dbl)
                n1704 = case shown="True" w2598 {
                  tunnel: w2597 -> [w2604 w2618]
                  tunnel: "Chemyx Syringe Pump Serial Port" -> [w2601 w2617]
                  frame False {
                    n1705 = flat-sequence {
                      tunnel: w2601 -> [w2605]
                      tunnel: [w2605] -> w2602
                      tunnel: w2604 -> [_]
                      tunnel: [w2608] -> w2603
                      tunnel: w2602 -> [w2608]
                      tunnel: w2603 -> [w2609]
                      tunnel: [w2609] -> w2599
                      tunnel: [w2611] -> w2600
                      tunnel: w2599 -> [w2611]
                      tunnel: w2600 -> [w2613]
                      frame #0 {
                        n1706 = call "Write to pump.vi"("string"="enter pump3", "VISA resource name"=w2605) -> ()  [unwired: 1 out]
                      }
                      frame #1 {
                        n1707 = local read "Pump pause delay (ms)"() -> (w2607:u32)
                        n1708 = Wait (ms)(milliseconds to wait=w2607) -> ()  [unwired: 1 out]
                      }
                      frame #2 {
                        n1709 = call "Write to pump.vi"("string"="stop", "VISA resource name"=w2609) -> ()  [unwired: 1 out]
                      }
                      frame #3 {
                        n1710 = Wait (ms)(milliseconds to wait=u32 0) -> ()  [unwired: 1 out]
                      }
                      frame #4 {
                        n1711 = call "Write to pump.vi"("string"="stop", "VISA resource name"=w2613) -> ()  [unwired: 1 out]
                      }
                    }
                  }
                  frame True {
                    n1712 = flat-sequence {
                      tunnel: w2617 -> [w2627]
                      tunnel: w2618 -> [w2622]
                      tunnel: w2618 -> [w2629]
                      tunnel: w2617 -> [w2630]
                      tunnel: [w2630] -> w2616
                      tunnel: [w2633] -> w2615
                      tunnel: w2616 -> [w2633]
                      tunnel: w2615 -> [w2634]
                      frame #0 {
                        n1713 = local read "All Pump Parameters"() -> (w2621:T10)
                        n1714 = Unbundle By Name(w2621) -> ("Pump 3"=w2628:T48)
                        n1715 = call "Set pump parameters.vi"("Pump write delay (ms)"=w2622, "Volume (uL)"="Ch 3 Inject Volume (uL)", "Rate (uL/h)"="Ch 3 Inject Rate (ul/h)", "Units"=4.0, "Pump #"=3.0, "Pump Parameters In"=w2628, "VISA resource name"=w2627) -> ("Pump Parameters Out"=w2620:T48)  [unwired: 3 in]
                        n1716 = Bundle By Name(cluster=w2621, "Pump 3"=w2620) -> (w2619:T10)
                        n1717 = local write "All Pump Parameters"(w2619) -> ()
                      }
                      frame #1 {
                        n1718 = Wait (ms)(milliseconds to wait=w2629) -> ()  [unwired: 1 out]
                      }
                      frame #2 {
                        n1719 = call "Write to pump.vi"("string"="start", "VISA resource name"=w2630) -> ()  [unwired: 1 out]
                      }
                      frame #3 {
                        n1720 = Wait (ms)(milliseconds to wait=u32 500) -> ()  [unwired: 1 out]
                      }
                      frame #4 {
                        n1721 = call "Write to pump.vi"("string"="start", "VISA resource name"=w2634) -> ()  [unwired: 1 out]
                      }
                    }
                  }
                }
              }
              frame True {
                n1722 = case shown="False" w2639 {
                  tunnel: w2640 -> [w2652 w2659]
                  frame False {
                    n1723 = flat-sequence {
                      tunnel: w2652 -> [w2654]
                      frame #0 {
                        n1724 = local write "Flushing P3"(FALSE ("Flushing P3")) -> ()
                        n1725 = Concatenate Strings("stop" ("string"), "\r") -> (w2656:string)
                        n1726 = VISA Write(VISA resource name=w2654, write buffer=w2656) -> ()  [unwired: 1 in, 3 out]
                      }
                      frame #1 {
                        n1727 = property on="Clear Volume P3" class="Bool (strict)"("Val(Sgnl)"=TRUE ("Value (Signaling)")) -> ()  [unwired: 2 in, 2 out]
                      }
                    }
                  }
                  frame True {
                    n1728 = local read "Normal Flow Rate (ul/h) P3"() -> (w2660:dbl)
                    n1729 = Number To Decimal String(number=w2660) -> (decimal integer string=w2666:string)  [unwired: 1 in]
                    n1730 = Concatenate Strings("irate  " ("string"), w2666, " u/h" ("string"), "\r") -> (w2664:string)
                    n1731 = VISA Write(VISA resource name=w2659, write buffer=w2664) -> (VISA resource name out=w2662:refnum<visa-resource-name>)  [unwired: 1 in, 2 out]
                    n1732 = Concatenate Strings("irun" ("string"), "\r") -> (w2668:string)
                    n1733 = VISA Write(VISA resource name=w2662, write buffer=w2668) -> ()  [unwired: 1 in, 3 out]
                  }
                }
                n1734 = local read "Save Event Log?"() -> (w2637:bool)
                n1735 = local read "Saving..."() -> (w2638:bool)
                n1736 = And(x=w2638, y=w2637) -> (x .and. y?=w2636:bool)
                n1737 = case shown="True" w2636 {
                  tunnel: w2639 -> [_ w2647]
                  frame False {
                  }
                  frame True {
                    n1738 = local read "Normal Flow Rate (ul/h) P3"() -> (w2641:dbl)
                    n1739 = Number To Decimal String(number=w2641) -> (decimal integer string=w2643:string)  [unwired: 1 in]
                    n1740 = Concatenate Strings("on, flow rate", w2643) -> (w2642:string)
                    n1741 = local read "log file ref"() -> (w2646:refnum<file>)
                    n1742 = Select(t=w2642, s=w2647, f="off") -> (s? t:f=w2648:string)
                    n1743 = local read "Time (s)"() -> (w2645:dbl)
                    n1744 = Concatenate Strings("pump 3 ", w2648) -> (w2650:string)
                    n1745 = call "write to event log.vi"("log file ref"=w2646, "time"=w2645, "input string"=w2650) -> ()  [unwired: 8 in]
                  }
                }
              }
            }
          }
          frame Enabled {
          }
        }
      }
      event "Inject Pump 2": Value Change {
        n1746 = event-data() -> ()  [unwired: 7 out]
        n1747 = local read "Pump write delay (ms)"() -> (w2675:dbl)
        n1748 = local read "Chemyx Syringe Pump Serial Port"() -> (w2674:refnum<visa-resource-name>)
        n1749 = flat-sequence {
          tunnel: w2674 -> [w2699]
          tunnel: w2675 -> [w2695]
          tunnel: "Inject Pump 2" -> [_]
          tunnel: w2675 -> [w2701]
          tunnel: w2674 -> [w2702]
          frame #0 {
            n1750 = local read "All Pump Parameters"() -> (w2694:T10)
            n1751 = Multiply(x=60.0, y="Flush Center Ch Rate (ul/m)") -> (x*y=w2691:dbl)
            n1752 = Unbundle By Name(w2694) -> ("Pump 2"=w2700:T48)
            n1753 = call "Set pump parameters.vi"("Pump write delay (ms)"=w2695, "Volume (uL)"="Flush Center Ch Volume (uL)", "Rate (uL/h)"=w2691, "Units"=3.0, "Pump #"=2.0, "Pump Parameters In"=w2700, "VISA resource name"=w2699) -> ("Pump Parameters Out"=w2693:T48)  [unwired: 3 in]
            n1754 = Bundle By Name(cluster=w2694, "Pump 2"=w2693) -> (w2692:T10)
            n1755 = local write "All Pump Parameters"(w2692) -> ()
            n1756 = Add(x="Flush Center Ch Volume (uL)", y="Total Volume\nFlushed (uL)") -> (x+y=w2688:dbl)
            n1757 = local write "Total Volume\nFlushed (uL)"(w2688) -> ()
          }
          frame #1 {
            n1758 = Wait (ms)(milliseconds to wait=w2701) -> ()  [unwired: 1 out]
          }
          frame #2 {
            n1759 = call "Write to pump.vi"("string"="start", "VISA resource name"=w2702) -> ()  [unwired: 1 out]
          }
        }
        n1760 = local read "Save Event Log?"() -> (w2673:bool)
        n1761 = local read "Saving..."() -> (w2672:bool)
        n1762 = And(x=w2673, y=w2672) -> (x .and. y?=w2671:bool)
        n1763 = case shown="True" w2671 {
          tunnel: "Inject Pump 2" -> [_ w2682]
          frame False {
          }
          frame True {
            n1764 = local read "Flow rate (uL/h)"() -> (w2676:dbl)
